vi "Delete listbox.vi"(8 "error in (no error)":errorcluster, 11 "Turnos in":refnum<class "Turnos.lvclass">) -> (0 "error out":errorcluster, 3 "Turnos out":refnum<class "Turnos.lvclass">)   [LabVIEW 2020, in "Turnos.lvlib" / "Turnos.lvclass"]
uses:
  Turnos.lvclass
  Turnos.lvclass/Turnos.ctl
  <vilib>/drjdpowell/SQLite Library/SQL Connection/Open (path).vi
  <vilib>/drjdpowell/SQLite Library/SQL Connection/Open (string).vi
  <vilib>/AdvancedString/Path To Command Line String.vi
  <vilib>/drjdpowell/SQLite Library/SQL Connection/Execute SQL.vi
  <vilib>/drjdpowell/SQLite Library/SQL Connection/Connection.lvclass
  <vilib>/drjdpowell/SQLite Library/SQLite.lvlib
panel:
  out "Servicio Estatus":string[][](array[string])
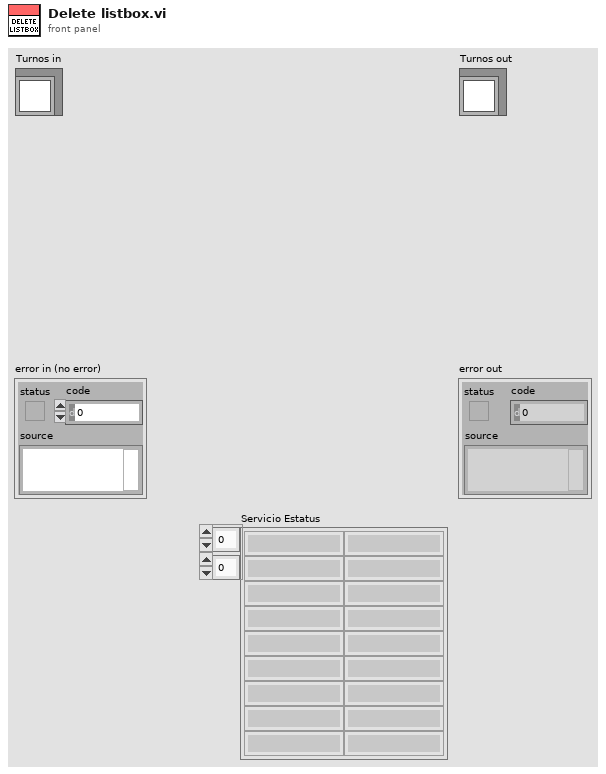
[diagram p1: front panel]
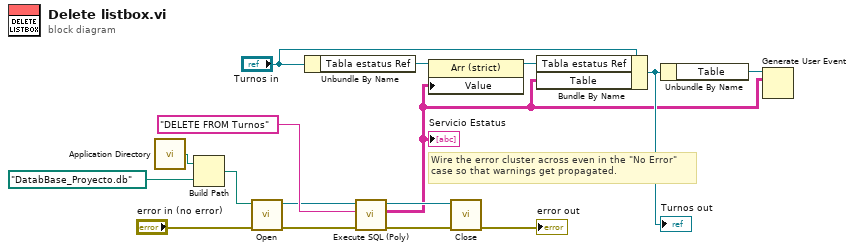
[diagram p0: block diagram]
diagram:
  # "Wire the error cluster across even in the \"No Error\"\ncase so that warnings get propagated."
  n1 = call <vilib>:"Application Directory.vi"() -> ("Application Directory"=w11:path)
  n2 = Build Path(base path=w11, name or relative path=path "DatabBase_Proyecto.db") -> (appended path=w9:path)
  n3 = call-poly <vilib>:"Open.vi"("error in (no error)"="error in (no error)", "db file"=w9) -> ("error out"=w13:errorcluster, "SQLite Connection"=w8:refnum<class "Connection.lvclass">)  [unwired: 8 in]
  n4 = Unbundle By Name("Turnos in") -> ("Tabla estatus Ref"=w5:refnum<vi>)
  n5 = call-poly <vilib>:"Execute SQL (Poly).vi"("error in (no error)"=w13, "SQL"="DELETE FROM Turnos", "SQLite Connection in"=w8) -> ("error out"=w14:errorcluster, "Result Set"=w1:string[][], "SQLite Connection"=w7:refnum<class "Connection.lvclass">)  [unwired: 5 in, 1 out]
  "Servicio Estatus" <- w1
  n6 = property class="Arr (strict)"(reference=w5, "Value"=w1) -> (reference out=w4:refnum<vi>)  [unwired: 1 in, 1 out]
  n7 = call-dynamic "Close.vi"("error in (no error)"=w14, "SQLite Connection in"=w7) -> ("error out"=→"error out":errorcluster)  [unwired: 9 in]
  n8 = Bundle By Name(cluster="Turnos in", "Tabla estatus Ref"=w4, "Table"=w1) -> (w3:refnum<class "Turnos.lvclass">)
  "Turnos out" <- w3
  n9 = Unbundle By Name(w3) -> ("Table"=w2:refnum<user-event>)
  n10 = Generate User Event(user event=w2, event data cluster=w1) -> ()  [unwired: 2 in, 2 out]
